vi "LVITX R+coord Commands.vi"(0 "2D wavename":string="R060731ASBDHS_0022", 5 "X wavename":string="0022x", 7 "Y wavename":string="0022y", 9 "N wavename":string="0022N", 11 "Ns wavename":string="0022Ns", 13 "input string":string="SetScale/I x -2.5e-05,2.5e-05,\"m\",  '#wave2D#';DelayUpdate\nSetScale/I y -2.5e-05,2.5e-05,\"m\",  '#wave2D#'\n\nDisplay;AppendImage '#wave2D#'\nModifyGraph width=288,height={Aspect,1}\n\nAppendToGraph '#waveY#' vs '#waveX#'\nModifyGraph mode=4,textMarker('#waveY#')={'#waveNs#',\"default\",0,0,0,0.00,0.00}\nModifyGraph mode=3,zColor('#waveY#')={'#waveN#',*,*,Rainbow,0}\n") -> (4 "result string":string="SetScale/I x -2.5e-05,2.5e-05,\"m\",  'R060731ASBDHS_0022';DelayUpdate\nSetScale/I y -2.5e-05,2.5e-05,\"m\",  'R060731ASBDHS_0022'\n\nDisplay;AppendImage 'R060731ASBDHS_0022'\nModifyGraph width=288,height={Aspect,1}\n\nAppendToGraph '0022y' vs '0022x'\nModifyGraph mode=4,textMarker('0022y')={'0022Ns',\"default\",0,0,0,0.00,0.00}\nModifyGraph mode=3,zColor('0022y')={'0022N',*,*,Rainbow,0}\n")   [LabVIEW 2011]
panel:
  # "Display;AppendImage R060731ASBDHS_0021\n# Delimited text load from \"cursor_R060731ASBDHS_0021.ibw.txt\"\n# LoadWave is unable to find column names on line 0\n# Data length: 20, waves: 0021x, 0021y, 0021N, 0021Ns\nSetScale/I x -2.5e-05,2.5e-05,\"m\", R060731ASBDHS_0021;DelayUpdate\nSetScale/I y -2.5e-05,2.5e-05,\"m\", R060731ASBDHS_0021\nAppendToGraph '0021y' vs '0021x'\nModifyGraph mode=4,textMarker('0021y')={'0021Ns',\"default\",0,0,0,0.00,0.00}\nModifyGraph mode=3,zColor('0021y')={'0021N',*,*,Rainbow,0}\nModifyGraph width=288,height={Aspect,1}"
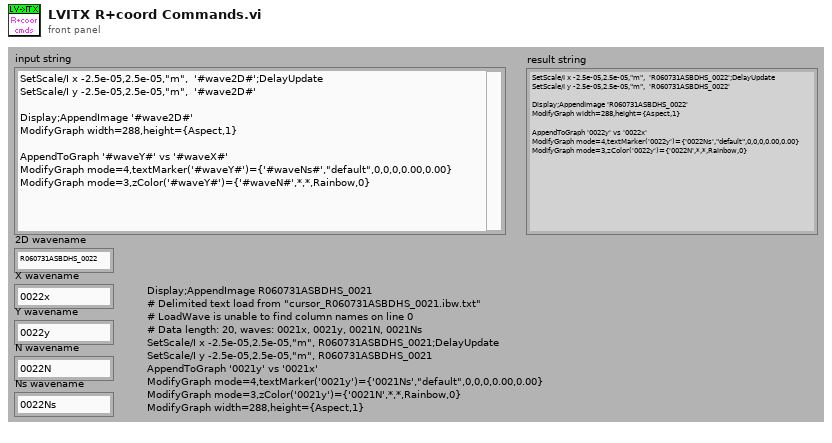
[diagram p1: front panel]
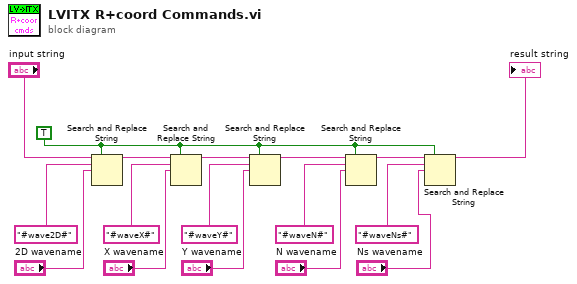
[diagram p0: block diagram]
diagram:
  w4 = TRUE ("replace all? (F)")
  n1 = Search and Replace String(replace all?=w4, input string="input string", search string="#wave2D#", replace string="2D wavename") -> (result string=w10:string)  [unwired: 1 in, 6 out]
  n2 = Search and Replace String(replace all?=w4, input string=w10, search string="#waveX#", replace string="X wavename") -> (result string=w12:string)  [unwired: 1 in, 6 out]
  n3 = Search and Replace String(replace all?=w4, input string=w12, search string="#waveY#", replace string="Y wavename") -> (result string=w5:string)  [unwired: 1 in, 6 out]
  n4 = Search and Replace String(replace all?=w4, input string=w5, search string="#waveN#", replace string="N wavename") -> (result string=w8:string)  [unwired: 1 in, 6 out]
  n5 = Search and Replace String(replace all?=w4, input string=w8, search string="#waveNs#", replace string="Ns wavename") -> (result string=→"result string":string)  [unwired: 1 in, 6 out]
